vi "Read handle.vi"(8 "error in (no error)":errorcluster, 11 "MultiUsrp in":refnum<class "MultiUsrp.lvclass">) -> (0 "error out":errorcluster, 2 "handle":dbl, 3 "MultiUsrp out":refnum<class "MultiUsrp.lvclass">)   [LabVIEW 2023, in "uhd.lvlib" / "MultiUsrp.lvclass"]
uses:
  <userlib>/uhd/MultiUsrp/MultiUsrp.lvclass
  <userlib>/uhd/MultiUsrp/MultiUsrp.lvclass/MultiUsrp.ctl
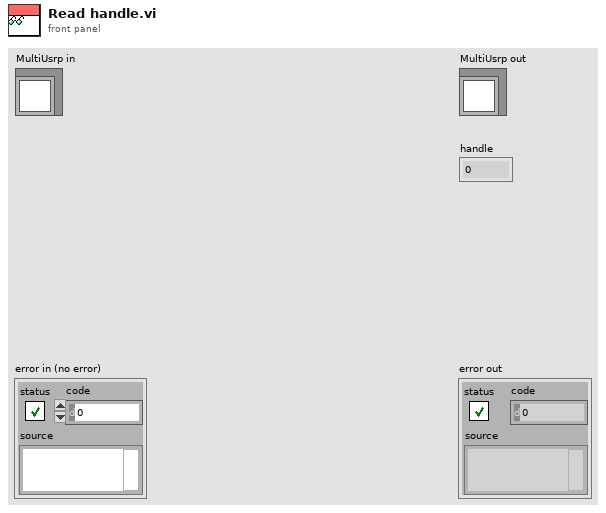
[diagram p1: front panel]
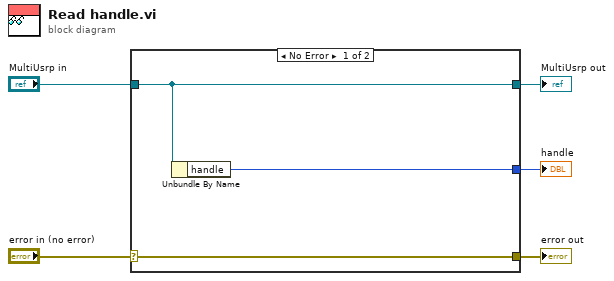
[diagram p0: block diagram]
diagram:
  n1 = case shown="No Error" "error in (no error)" {
    selector: "error in (no error)" -> [w8 w9]
    tunnel: [w8 w9] -> w4
    tunnel: [w7 w10] -> w2
    tunnel: "MultiUsrp in" -> [w7 w10]
    tunnel: [w6 _] -> w1
    frame No Error {
      n2 = Unbundle By Name(w7) -> ("handle"=w6:u64)
    }
    frame Error {
    }
  }
  "error out" <- w4
  "MultiUsrp out" <- w2
  "handle" <- w1
